vi "Read Waveform.vi"(8 "error in (no error)":errorcluster, 10 "Channel":T1, 11 "PicoScope 3000a in":refnum<class "PicoScope 3000a.lvclass">) -> (0 "error out":errorcluster, 2 "Waveform":waveform(dbl)(graph), 3 "PicoScope 3000a out":refnum<class "PicoScope 3000a.lvclass">)   [LabVIEW 2018, in "PicoScope 3000a.lvlib" / "PicoScope 3000a.lvclass"]
doc: "This Override method is used to initiate waveform acquisition. Select targeted channel at the 'Channel' control and output waveform data to the 'Waveform' indicator."
uses:
  PicoScope 3000a.lvclass
  LWS SLA-070/Distro/Projects/12170 Luminar LWS Base/Source/PPLs/Oscilloscope.lvlibp/Custom Controls/Analog Channels.ctl
  PicoScope 3000a.lvclass/PicoScope 3000a.ctl
  <instrlib>/PicoScope/PicoScope.lvlib
  LWS SLA-070/Distro/Projects/12170 Luminar LWS Base/Source/PPLs/Oscilloscope.lvlibp
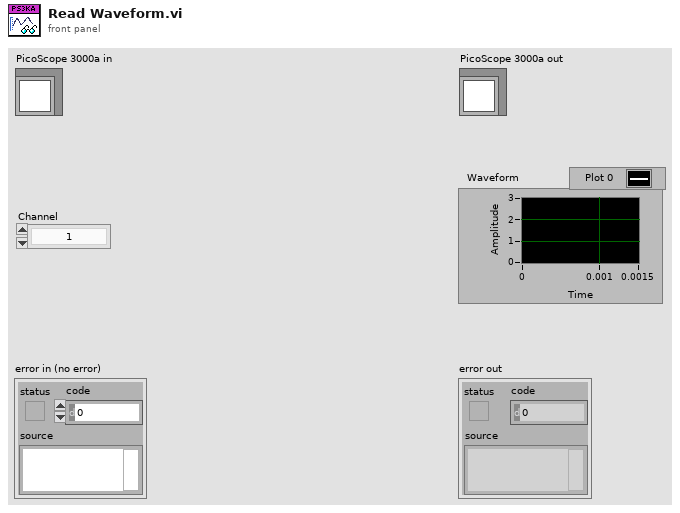
[diagram p1: front panel]
types:
  T1 = typedef "Oscilloscope.lvlibp/Analog Channels.ctl" = enum16{"1", "2", "3", "4", "5", "6", "7", "8", "9", "10", "11", "12", "13", "14", "15", "16"}
  T2 = cluster{"Driver Version":string, "USB Version":string, "Hardware":string, "Variant":string, "Batch and Serial":string, "Cal Date":string, "Kernel Version":string, "Digital HW Version":string, "Analogue HW Version":string, "MSO":bool, "Number of channels":i16}
  T3 = cluster{"preTriggerSamples":u32, "postTriggerSamples":u32, "timebase":u32, "Down-Sample Mode":i32, "Down Sample Ratio":u32}
  T4 = cluster{"Channel":enum16{"CH. A", "CH. B", "CH. C", "CH. D"}, "Range":u32}[]
  T5 = cluster{"Channel D Buffer":i16[], "Channel C Buffer":i16[], "Channel B Buffer":i16[], "Channel A Buffer":i16[], "Port 0  Buffer ":i16[], "Port 1 Buffer ":i16[]}
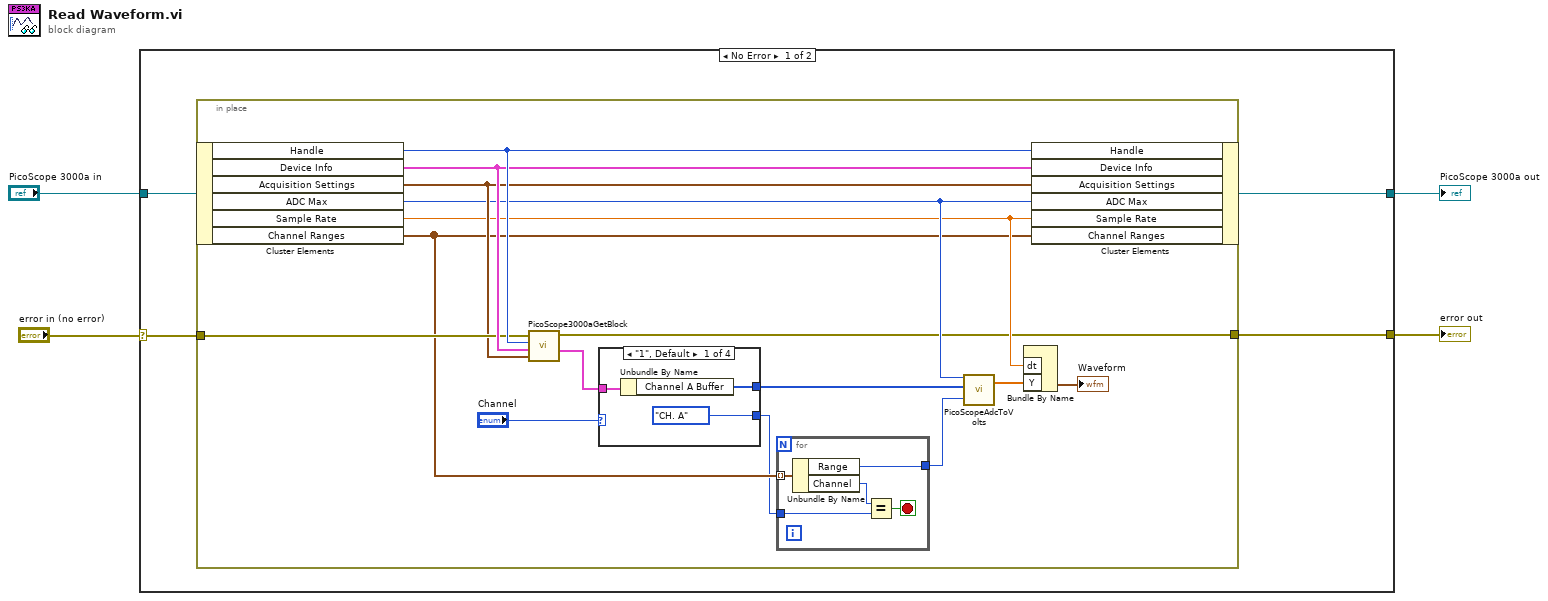
[diagram p0: block diagram]
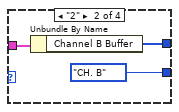
[diagram p2: hidden frame]
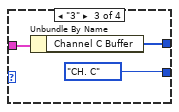
[diagram p3: hidden frame]
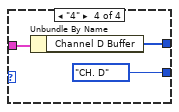
[diagram p4: hidden frame]
diagram:
  n1 = case shown="No Error" "error in (no error)" {
    selector: "error in (no error)" -> [w7 w41]
    tunnel: "PicoScope 3000a in" -> [w8 w42]
    tunnel: [w6 w41] -> w2
    tunnel: [w5 w42] -> w1
    frame No Error {
      n2 = in-place {
        in-place-border: w7 -> [w21]
        in-place-border: [w12] -> w6
        n3 = in-place-cluster #1(w8) -> ("Handle"=w23:i16, "Device Info"=w22:T2, "Acquisition Settings"=w20:T3, "ADC Max"=w16:i16, "Sample Rate"=w13:sgl, "Channel Ranges"=w11:T4)
        n4 = call <instrlib>:"PicoScope3000aGetBlock.vi"("error in"=w21, "handle in"=w23, "Acquisition Settings"=w20, "Device Info"=w22) -> ("error out"=w12:errorcluster, "Buffers (Max or non-aggregated)"=w18:T5)  [unwired: 1 in, 4 out]
        n5 = case shown="\"1\", Default" "Channel" {
          tunnel: w18 -> [w31 w34 w37 w40]
          tunnel: [w30 w33 w36 w39] -> w17
          tunnel: [enum16{"CH. A", "CH. B", "CH. C", "CH. D"}."CH. A" ("Channel") enum16{"CH. A", "CH. B", "CH. C", "CH. D"}."CH. B" ("Channel") enum16{"CH. A", "CH. B", "CH. C", "CH. D"}."CH. C" ("Channel") enum16{"CH. A", "CH. B", "CH. C", "CH. D"}."CH. D" ("Channel")] -> w10
          frame "1", Default {
            n6 = Unbundle By Name(w31) -> ("Channel A Buffer"=w30:i16[])
          }
          frame "2" {
            n7 = Unbundle By Name(w34) -> ("Channel B Buffer"=w33:i16[])
          }
          frame "3" {
            n8 = Unbundle By Name(w37) -> ("Channel C Buffer"=w36:i16[])
          }
          frame "4" {
            n9 = Unbundle By Name(w40) -> ("Channel D Buffer"=w39:i16[])
          }
        }
        n10 = for {
          tunnel: w11 -> [w28] mode=indexing
          tunnel: [w25] -> w9
          tunnel: w10 -> [w24]
          stop <- w26 stop-if-true
          n11 = Unbundle By Name(w28) -> ("Range"=w25:u32, "Channel"=w27:enum16{"CH. A", "CH. B", "CH. C", "CH. D"})
          n12 = Equal?(x=w27, y=w24) -> (x = y?=w26:bool)
        }
        n13 = call <instrlib>:"PicoScopeAdcToVolts.vi"("Max_adc"=w16, "Range Index"=w9, "Data"=w17) -> ("Data (Volts)"=w15:dbl[])
        n14 = Bundle By Name("dt"=w13, "Y"=w15) -> (→"Waveform":waveform(dbl))  [unwired: 1 in]
        n15 = in-place-cluster #1("Handle"=w23, "Device Info"=w22, "Acquisition Settings"=w20, "ADC Max"=w16, "Sample Rate"=w13, "Channel Ranges"=w11) -> (w5:refnum<class "PicoScope 3000a.lvclass">)
      }
    }
    frame Error {
    }
  }
  "error out" <- w2
  "PicoScope 3000a out" <- w1
